vi "FG-Resources.vi"(8 "error in":errorcluster, 11 "Config. params. ref. in":refnum<data-value>) -> (0 "error IO":errorcluster, 2 "Succes?":bool, 3 "Config. params. ref.":refnum<data-value>)   [LabVIEW 2013, in "CameraVision.lvlib" / "CV-Configuration.lvclass"]
uses:
  CV-Configuration.lvclass
  CV-Configuration.lvclass/CV-Configuration.ctl
  Read Framegrabber DLL file.vi
  Read BoardHandle.vi
  Read Camport array.vi
  Read Image sizes.vi
  Read Framegrabber buffer.vi
  Write DMA adresses.vi
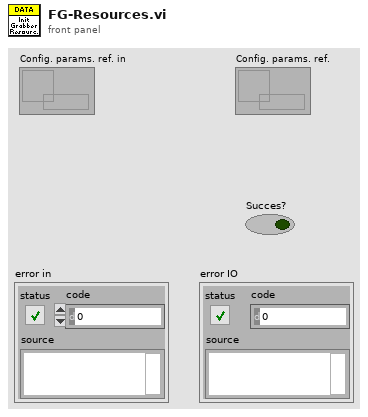
[diagram p1: front panel]
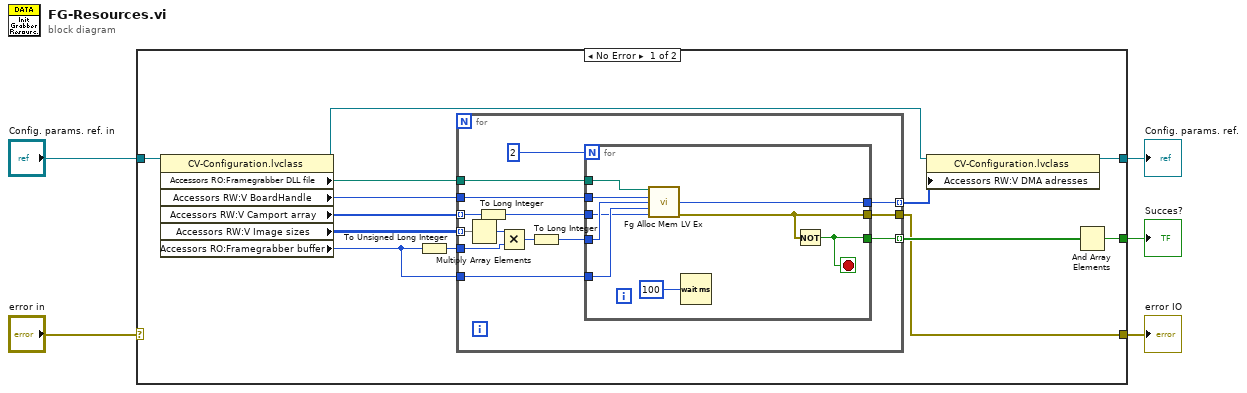
[diagram p0: block diagram]
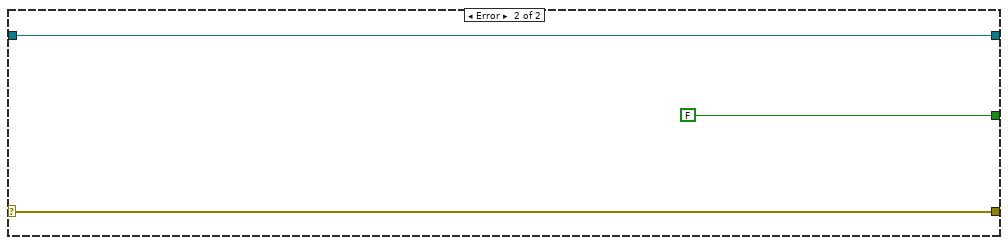
[diagram p2: hidden frame]
diagram:
  n1 = case shown="No Error" "error in" {
    selector: "error in" -> [_ w44]
    tunnel: [w7 w44] -> w5
    tunnel: [w17 FALSE] -> w3
    tunnel: "Config. params. ref. in" -> [w15 w42]
    tunnel: [w10 w42] -> w1
    frame No Error {
      n2 = property class="CV-Configuration.lvclass"(reference=w15) -> (reference out=w11:refnum<data-value>, "Accessors RO:Framegrabber DLL file"=w8:path, "Accessors RW:V BoardHandle"=w13:u64, "Accessors RW:V Camport array"=w14:u32[], "Accessors RW:V Image sizes"=w12:u32[][], "Accessors RO:Framegrabber buffer"=w6:i32)  [unwired: 1 in, 1 out]
      n3 = To Unsigned Long Integer(number=w6) -> (unsigned 32bit integer=w16:u32)
      n4 = for {
        tunnel: w16 -> [w29]
        tunnel: [w32] -> w18 mode=indexing
        tunnel: w14 -> [w27] mode=indexing
        tunnel: w13 -> [w26]
        tunnel: w8 -> [w25]
        tunnel: w12 -> [w24] mode=indexing
        tunnel: w6 -> [w21]
        tunnel: [w20] -> w9 mode=indexing
        tunnel: [w19] -> w7
        n5 = Multiply Array Elements(1:w24) -> (0:w30:u32)
        n6 = To Long Integer(number=w27) -> (32bit integer=w23:i32)
        n7 = Multiply(x=w30, y=w29) -> (x*y=w28:u32)
        n8 = To Long Integer(number=w28) -> (32bit integer=w22:i32)
        n9 = for {
          N: 2 -> [_]
          tunnel: [w37] -> w32
          tunnel: w21 -> [w38]
          tunnel: w22 -> [w39]
          tunnel: w23 -> [w35]
          tunnel: w26 -> [w36]
          tunnel: w25 -> [w40]
          tunnel: [w34] -> w20
          tunnel: [w33] -> w19
          stop <- w37 stop-if-true
          n10 = call <userlib>:"Fg Alloc Mem LV Ex.vi"("dll path in"=w40, "FgAddr"=w36, "Size"=w39, "Nr_Of_Buf"=w38, "CamPort"=w35) -> ("function return"=w34:i64, "error out"=w33:errorcluster)  [unwired: 8 in, 1 out]
          n11 = Wait (ms)(milliseconds to wait=u32 100) -> ()  [unwired: 1 out]
          n12 = Not(x=w33) -> (.not. x?=w37:bool)
        }
      }
      n13 = property class="CV-Configuration.lvclass"(reference=w11, "Accessors RW:V DMA adresses"=w9) -> (reference out=w10:refnum<data-value>)  [unwired: 1 in, 1 out]
      n14 = And Array Elements(Boolean array=w18) -> (logical AND=w17:bool)
    }
    frame Error {
    }
  }
  "error IO" <- w5
  "Succes?" <- w3
  "Config. params. ref." <- w1
